vi "BRig_dataExp_Cue2Switch_Prob_1B.vi"() -> (2 "output_Cue2Switch_Prob_1B":i32)   [LabVIEW 2014]
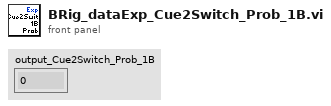
[diagram p1: front panel]
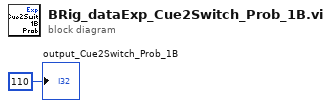
[diagram p0: block diagram]
diagram:
  "output_Cue2Switch_Prob_1B" <- 110 ("output_iBlock")
